vi "InsertData.vi"(8 "error in (no error)":errorcluster, 10 "Data Cluster":variant, 11 "object in":refnum<class "TableLogger_Actor.lvclass">) -> (0 "error out":errorcluster, 3 "object out":refnum<class "TableLogger_Actor.lvclass">)   [LabVIEW 2014, in "TableLogger_Actor.lvlib" / "TableLogger_Actor.lvclass"]
uses:
  TableLogger_Actor.lvclass
panel:
  # "Connector Pane"
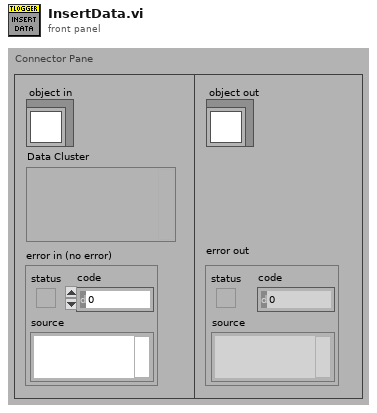
[diagram p1: front panel]
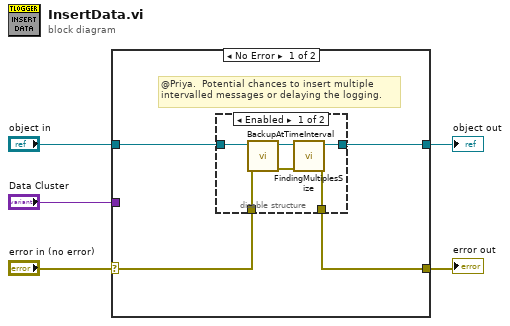
[diagram p0: block diagram]
diagram:
  n1 = case shown="No Error" "error in (no error)" {
    selector: "error in (no error)" -> [w7 w19]
    tunnel: [w8 w19] -> w4
    tunnel: [w9 w18] -> w2
    tunnel: "object in" -> [w6 w18]
    tunnel: "Data Cluster" -> [_ _]
    frame No Error {
      # "@Priya.  Potential chances to insert multiple\nintervalled messages or delaying the logging."
      n2 = disable-structure shown="Enabled" {
        disable-tunnel: [w15 w17] -> w9
        disable-tunnel: [w14 w16] -> w8
        disable-tunnel: w7 -> [w13 w16]
        disable-tunnel: w6 -> [w11 w17]
        frame Enabled {
          n3 = call "BackupAtTimeInterval.vi"("error in (no error)"=w13, "object in"=w11) -> ("error out"=w12:errorcluster, "object out"=w10:refnum<class "TableLogger_Actor.lvclass">)  [unwired: 8 in]
          n4 = call "FindingMultiplesSize.vi"("error in (no error)"=w12, "TableLogger_Actor in"=w10) -> ("error out"=w14:errorcluster, "TableLogger_Actor out"=w15:refnum<class "TableLogger_Actor.lvclass">)  [unwired: 7 in, 1 out]
        }
        frame Disabled {
        }
      }
    }
    frame Error {
    }
  }
  "error out" <- w4
  "object out" <- w2
